vi "Show Reservation Errors.vi"(10 "Errors":errorcluster[](array[cluster]), 11 "Aliases":string[](array[string])) -> ()   [LabVIEW 2020]
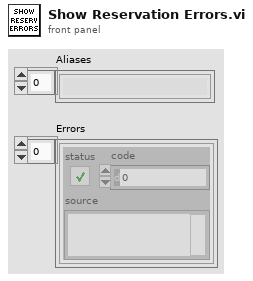
[diagram p1: front panel]
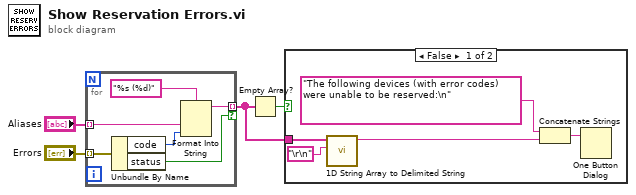
[diagram p0: block diagram]
diagram:
  n1 = for {
    tunnel: "Aliases" -> [w7] mode=indexing
    tunnel: "Errors" -> [w9] mode=indexing
    tunnel: [w6] -> w2 mode=indexing if=w5
    n2 = Unbundle By Name(w9) -> ("code"=w8:i32, "status"=w5:bool)
    n3 = Format Into String(format string="%s (%d)", w7, w8) -> (resulting string=w6:string)  [unwired: 2 in, 1 out]
  }
  n4 = Empty Array?(array=w2) -> (empty?=w1:bool)
  n5 = case shown="False" w1 {
    tunnel: w2 -> [w15 _]
    frame False {
      n6 = call <vilib>:"1D String Array to Delimited String.vi"("delimiter"="\r\n", "string array"=w15) -> ("delimited string"=w13:string)  [unwired: 9 in]
      n7 = Concatenate Strings("The following devices (with error codes) were unable to be reserved:\n", w13) -> (w11:string)
      n8 = One Button Dialog(message=w11) -> ()  [unwired: 1 in, 1 out]
    }
    frame True {
    }
  }
